vi "Keithley_Standalone_RS-232.vi"() -> ()   [LabVIEW 2013]
uses:
  subVIs/Current_Range_Control.ctl
  <vilib>/Utility/file.llb/Write To Spreadsheet File (DBL).vi
panel:
  out "Scan Number":i32
  in  "Current Range Ch 2":T1 items=["Autorange", "+/- 20 mikroA", "+/- 2 mikroA", "+/- 200 nA", "+/- 20 nA", "+/- 2 nA"]
  in  "Current Range Ch 1":T1 items=["Autorange", "+/- 20 mikroA", "+/- 2 mikroA", "+/- 200 nA", "+/- 20 nA", "+/- 2 nA"]
  out "Standard Error":dbl[](array[numeric])
  in  "1D Array Order":i32[](array[numeric])
  out "Chart 2":cluster{"Time Array OUT":dbl[], dbl[]}(graph)
  out "Chart 1":cluster{"Time Array OUT":dbl[], dbl[]}(graph)
  in  "Invert Ch 2":bool
  in  "Invert Ch 1":bool
  out "t_loop":u32
  out "dumped data (%)":dbl
  out "dumped data":i32
  in  "Cluster":T2={"Baudrate (9600)"=57600, "Data Bits (8)"=8, "Parity (None)"=0, "Stop Bits (1)"=10, "Flow Control (None)"=0, "End Mode for Reads (TermChar)"=2} {"End Mode for Reads (TermChar)" items=["None", "Last Bit", "TermChar"]; "Flow Control (None)" items=["None", "XON/XOFF", "RTS/CTS", "XON/XOFF & RTS/CTS", "DTR/DSR", "XON/XOFF & DTR/DSR"]; "Stop Bits (1)" items=["1.0"=10, "1.5"=15, "2.0"=20]; "Parity (None)" items=["None", "Odd", "Even", "Mark", "Space"]; "Baudrate (9600)" items=["300"=300, "600"=600, "1200"=1200, "2400"=2400, "4800"=4800, "9600"=9600, "19200"=19200, "38400"=38400, "57600"=57600, "115200"=115200]}
  in  "VISA resource name":refnum<visa-resource-name>="COM1"
  out "SD Keithley":dbl[](array[numeric])
  out "Mean Keithley":dbl[](array[numeric])
  out "buffer":string
  out "use data":bool
  out "Status":i32 format="%.0b"
  in  "Stop Keithley":bool
  in  "error in (no error)":errorcluster
  out "error out":errorcluster
  # "file structure:     column 1      column 2       column 3\n                              time (s)         Ch 1 (amp)     Ch 2 (amp)"
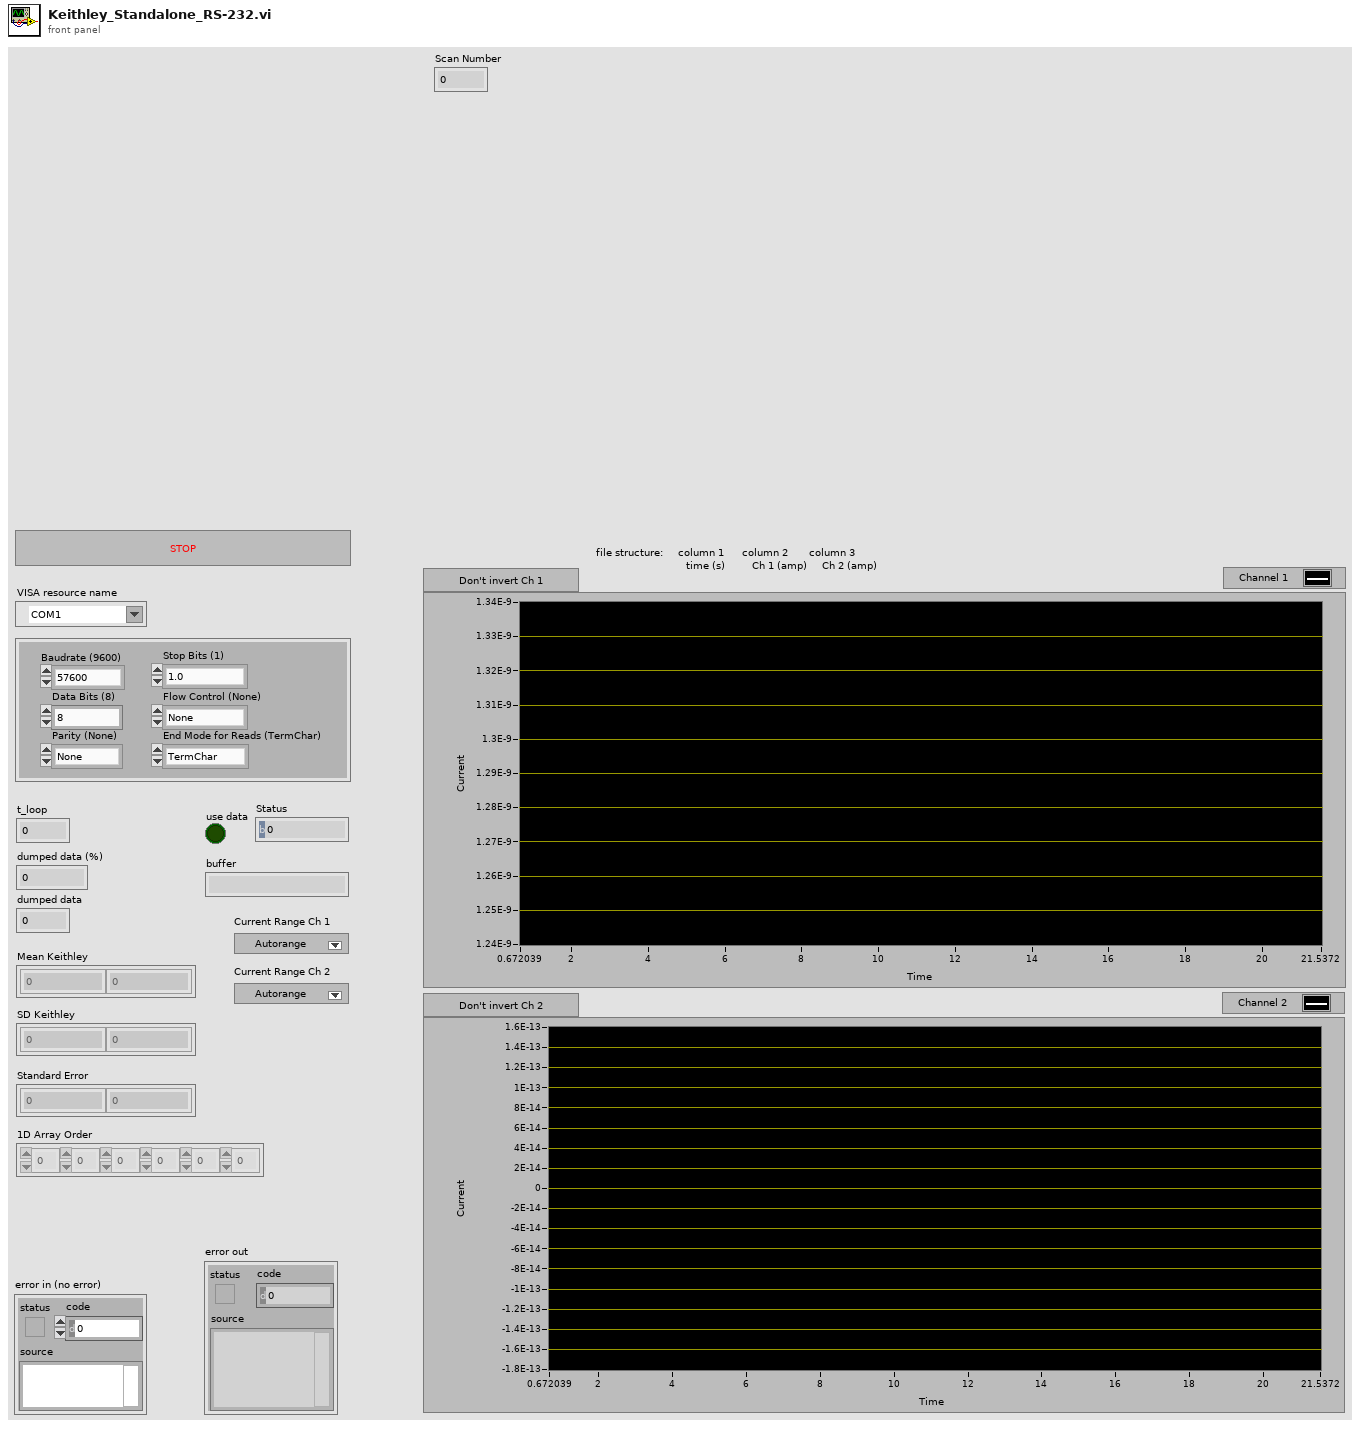
[diagram p1: front panel]
types:
  T1 = typedef "Current_Range_Control.ctl" = u16
  T2 = cluster{"Baudrate (9600)":u32, "Data Bits (8)":u16, "Parity (None)":u16, "Stop Bits (1)":u16, "Flow Control (None)":u16, "End Mode for Reads (TermChar)":u16}
  T3 = cluster{"Time Array OUT":dbl[], "Array OUT":dbl[]}
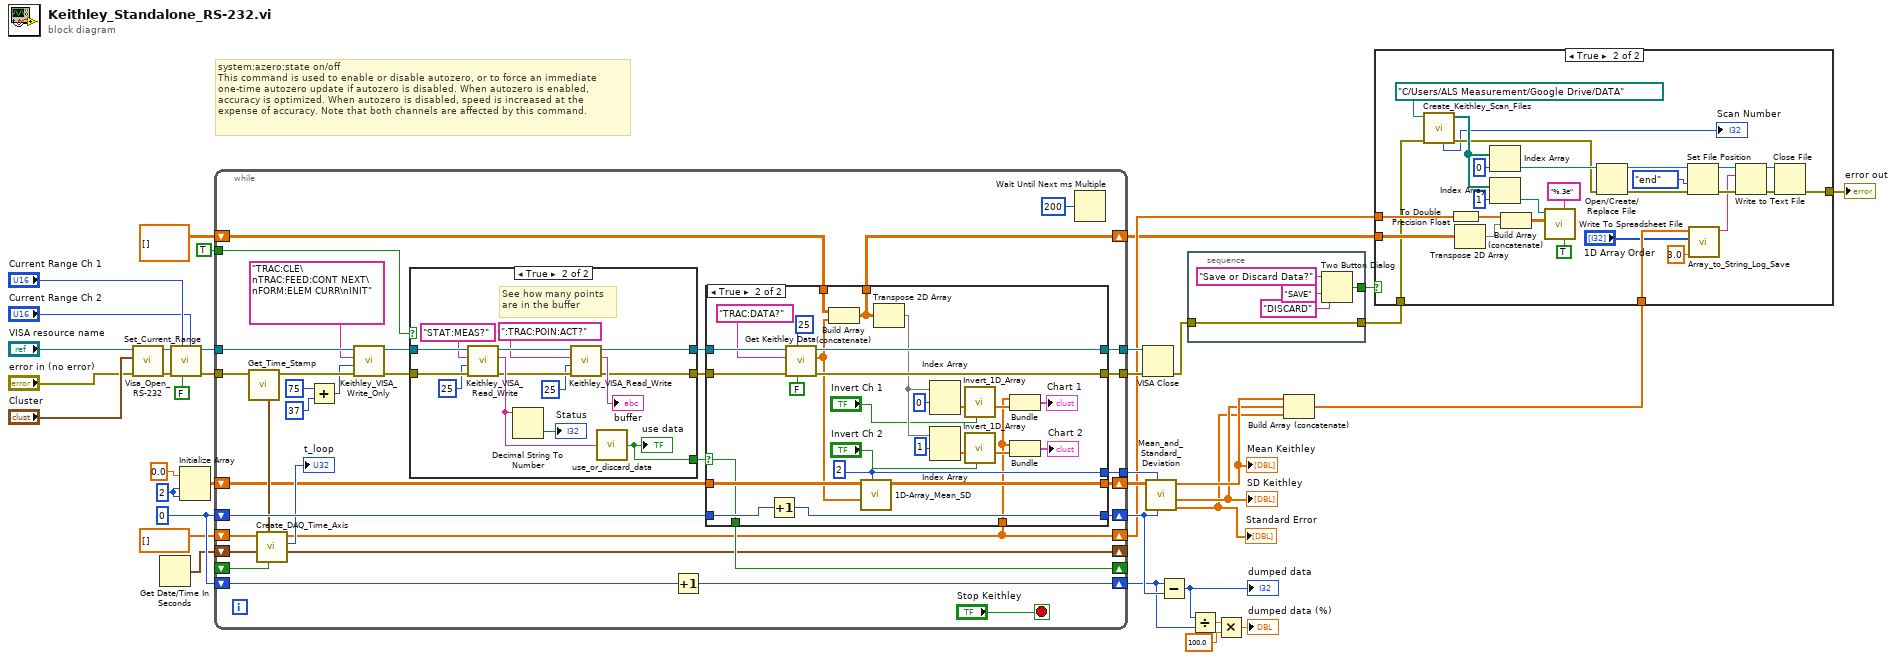
[diagram p0: block diagram]
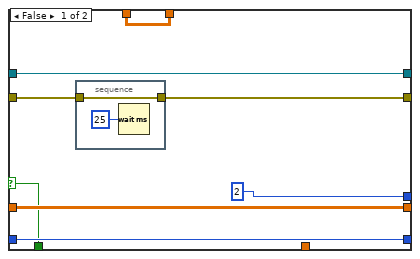
[diagram p3: hidden frame]
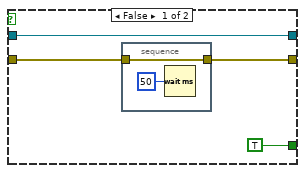
[diagram p4: hidden frame]
diagram:
  w24 = 0
  w37 = 2 ("dimension size")
  # "system:azero:state on/off\nThis command is used to enable or disable autozero, or to force an immediate\none-time autozero update if autozero is disabled. When autozero is enabled,\naccuracy is optimized. When autozero is disabled, speed is increased at the\nexpense of accuracy. Note that both channels are affected by this command."
  n1 = call "Visa_Open_RS-232.vi"("error in (no error)"="error in (no error)", "Cluster"="Cluster", "ComPort"="VISA resource name") -> ("error out"=w17:errorcluster, "VISA resource name out"=w15:refnum<visa-resource-name>)  [unwired: 7 in]
  n2 = Get Date/Time In Seconds() -> (seconds since 1Jan1904=w23:timestamp)
  n3 = call "Set_Current_Range.vi"("Current Range Ch 2"="Current Range Ch 2", "GPIB (t) / RS-232 (f)"=FALSE, "Current Range Ch 1"="Current Range Ch 1", "error in (no error)"=w17, "VISA resource name"=w15) -> ("error out"=w16:errorcluster, "VISA resource name out"=w18:refnum<visa-resource-name>)  [unwired: 5 in]
  n4 = Initialize Array(0.0 ("element"), w37, w37) -> (w36:dbl[][])
  n5 = while {
    tunnel: w18 -> [w61]
    tunnel: w16 -> [w55]
    tunnel: [w72] -> w20
    tunnel: [w56] -> w21
    tunnel: TRUE ("Check Completeness of Data (true)") -> [w71]
    shift-right: [w69] -> w34
    shift-left: w36 -> [w43]
    tunnel: [w68] -> w35
    shift-right: [w66] -> w30
    shift-left: w24 -> [w67]
    shift-right: [w63] -> w28
    shift-left: w24 -> [w64]
    shift-right: [w40] -> w9
    shift-left: dbl[] [] ("Time Array OUT") -> [w52]
    shift-right: [w41] -> w8
    shift-left: dbl[][] [] -> [w42]
    shift-right: [w50] -> _
    shift-left: w23 -> [w51]
    shift-right: [w53] -> _
    shift-left: _ -> [w49]
    stop <- "Stop Keithley" stop-if-true
    n6 = call "Get_Time_Stamp.vi"("error in"=w55) -> ("error out"=w54:errorcluster, "current time"=w47:timestamp)  [unwired: 9 in]
    n7 = call "Create_DAQ_Time_Axis.vi"("NOT [Last Data Point Dumped?]"=w49, "Time Stamp Current Iteration"=w47, "Time Stamp Last Iteration"=w51, "Time Array IN"=w52) -> ("Time Stamp Current Iteration"=w50:timestamp, "Loop Time (ms)"=→"t_loop":u32, "Time Array OUT"=w40:dbl[])  [unwired: 5 in]
    n8 = Add(x=u32 75 ("milliseconds to wait"), y=u32 37) -> (x+y=w45:u32)
    n9 = call "Keithley_VISA_Write_Only.vi"("error in (no error)"=w54, "milliseconds to wait"=w45, "command"="TRAC:CLE\nTRAC:FEED:CONT NEXT\nFORM:ELEM CURR\nINIT", "VISA resource name"=w61) -> ("error out"=w59:errorcluster, "VISA resource name out"=w60:refnum<visa-resource-name>)  [unwired: 6 in]
    n10 = case shown="True" w71 {
      tunnel: w60 -> [w114 w128]
      tunnel: w59 -> [w112 w129]
      tunnel: [w114 w119] -> w70
      tunnel: [TRUE w117] -> w62
      tunnel: [w111 w118] -> w65
      frame False {
        n11 = stacked-sequence {
          tunnel: w112 -> [w116]
          tunnel: [w116] -> w111
          frame #0 {
            n12 = Wait (ms)(milliseconds to wait=u32 50) -> ()  [unwired: 1 out]
          }
        }
      }
      frame True {
        # "See how many points\nare in the buffer"
        n13 = call "Keithley_VISA_Read_Write.vi"("error in (no error)"=w129, "milliseconds to wait"=u32 25, "command"="STAT:MEAS?" ("write buffer"), "VISA resource name"=w128) -> ("error out"=w124:errorcluster, "read buffer"=w125:string, "VISA resource name out"=w123:refnum<visa-resource-name>)  [unwired: 5 in]
        n14 = Decimal String To Number(string=w125) -> (number=→"Status":i32)  [unwired: 2 in, 1 out]
        n15 = call "Keithley_VISA_Read_Write.vi"("error in (no error)"=w124, "milliseconds to wait"=u32 25, "command"=":TRAC:POIN:ACT?" ("write buffer"), "VISA resource name"=w123) -> ("error out"=w118:errorcluster, "read buffer"=→"buffer":string, "VISA resource name out"=w119:refnum<visa-resource-name>)  [unwired: 5 in]
        n16 = call "use_or_discard_data.vi"("Status"=w125) -> ("use data"=w117:bool)
        "use data" <- w117
      }
    }
    n17 = Increment(x=w64) -> (x+1=w63:i32)
    n18 = case shown="True" w62 {
      selector: w62 -> [w73 w98]
      tunnel: [w77 w108] -> w72
      tunnel: [w75 w107] -> w56
      tunnel: w70 -> [w77 w110]
      tunnel: w65 -> [w76 w109]
      tunnel: w43 -> [w80 w106]
      tunnel: [w80 w105] -> w69
      tunnel: [2 ("N") w104] -> w68
      tunnel: w67 -> [w78 w103]
      tunnel: [w78 w102] -> w66
      tunnel: [w74 w95] -> w41
      tunnel: w42 -> [w74 w99]
      tunnel: [w73 w98] -> w53
      tunnel: w40 -> [_ w84]
      frame False {
        n19 = stacked-sequence {
          tunnel: w76 -> [w82]
          tunnel: [w82] -> w75
          frame #0 {
            n20 = Wait (ms)(milliseconds to wait=u32 25) -> ()  [unwired: 1 out]
          }
        }
      }
      frame True {
        w104 = 2 ("N")
        n21 = Increment(x=w103) -> (x+1=w102:i32)
        n22 = call "Get Keithley Data.vi"("GPIB = true, RS-232 = false"=FALSE, "wait after write (ms)"=u32 25 ("milliseconds to wait"), "error in (no error)"=w109, "Command"="TRAC:DATA?", "VISA resource name"=w110) -> ("error out"=w107:errorcluster, "Data"=w97:dbl[], "VISA resource name out"=w108:refnum<visa-resource-name>)  [unwired: 3 in, 1 out]
        n23 = Build Array (concatenate)(w99, w97) -> (w95:dbl[][])
        n24 = call "1D-Array_Mean_SD.vi"("N"=w104, "Data Array"=w97, "IN"=w106) -> ("OUT"=w105:dbl[][])  [unwired: 8 in]
        n25 = Transpose 2D Array(2D array=w95) -> (transposed array=w96:dbl[][])
        n26 = Index Array(array=w96, index (row)=0 ("index")) -> (element=w91:dbl[])  [unwired: 1 in]
        n27 = Index Array(array=w96, index (row)=1 ("index")) -> (element=w92:dbl[])  [unwired: 1 in]
        n28 = call "Invert_1D_Array.vi"("Invert?"="Invert Ch 1", "Array IN"=w91) -> ("Array OUT"=w86:dbl[])  [unwired: 9 in]
        n29 = call "Invert_1D_Array.vi"("Invert?"="Invert Ch 2", "Array IN"=w92) -> ("Array OUT"=w85:dbl[])  [unwired: 9 in]
        n30 = Bundle("Time Array OUT"=w84, "Array OUT"=w86) -> (→"Chart 1":T3)  [unwired: 1 in]
        n31 = Bundle("Time Array OUT"=w84, "Array OUT"=w85) -> (→"Chart 2":T3)  [unwired: 1 in]
      }
    }
    n32 = Wait Until Next ms Multiple(millisecond multiple=u32 200) -> ()  [unwired: 1 out]
  }
  n33 = VISA Close(VISA resource name=w20, error in (no error)=w21) -> (error out=w3:errorcluster)
  n34 = call "Mean_and_Standard_Deviation.vi"("Iterations"=w30, "Data Points"=w35, "2D array"=w34) -> ("Standard Error"=w11:dbl[], "Standard Deviation"=w12:dbl[], "Mean"=w13:dbl[])  [unwired: 6 in]
  "Mean Keithley" <- w13
  "SD Keithley" <- w12
  "Standard Error" <- w11
  n35 = Subtract(x=w28, y=w30) -> (x-y=w29:i32)
  "dumped data" <- w29
  n36 = stacked-sequence {
    tunnel: [w135] -> w1
    tunnel: w3 -> [w131]
    tunnel: [w131] -> w2
    frame #0 {
      n37 = Two Button Dialog(message="Save or Discard Data?", 1:"DISCARD" ("F button name (\"Cancel\")"), 2:"SAVE" ("T button name (\"OK\")")) -> (T button?=w135:bool)
    }
  }
  n38 = Divide(x=w29, y=w28) -> (x/y=w27:dbl)
  n39 = Multiply(x=w27, y=100.0) -> (x*y=→"dumped data (%)":dbl)
  n40 = Build Array (concatenate)(w13, w12, w11) -> (w10:dbl[])
  n41 = case shown="True" w1 {
    tunnel: w10 -> [_ w164]
    tunnel: w9 -> [_ w156]
    tunnel: w8 -> [_ w155]
    tunnel: [w136 w138] -> w4
    tunnel: w2 -> [w136 w137]
    frame False {
    }
    frame True {
      n42 = call "Create_Keithley_Scan_Files.vi"("error in (no error)"=w137, "base path"=path "C:/Users/ALS Measurement/Google Drive/DATA" ("file path (use dialog)")) -> ("error out"=w149:errorcluster, "Save Files Array"=w161:path[], "Scan Number"=→"Scan Number":i32)  [unwired: 5 in, 2 out]
      n43 = To Double Precision Float(number=w156) -> (double precision float=w158:dbl[])
      n44 = Transpose 2D Array(2D array=w155) -> (transposed array=w157:dbl[][])
      n45 = Index Array(array=w161, index=0) -> (element=w152:path)
      n46 = Index Array(array=w161, index=1) -> (element=w160:path)
      n47 = Build Array (concatenate)(w158, w157) -> (w159:dbl[][])
      n48 = call-poly <vilib>:"Write To Spreadsheet File.vi"("transpose? (no:F)"=TRUE, "format (%.3f)"="%.3e", "2D data"=w159, "file path (dialog if empty)"=w160) -> ()  [unwired: 4 in, 1 out]
      n49 = Open/Create/Replace File(file path (use dialog)=w152, error in=w149) -> (refnum out=w146:refnum<file>, error out=w148:errorcluster)  [unwired: 4 in, 1 out]
      n50 = Set File Position(refnum=w146, from (0:start)=enum16{"start", "end", "current"}."end", error in=w148) -> (refnum out=w145:refnum<file>, error out=w144:errorcluster)  [unwired: 1 in]
      n51 = call "Array_to_String_Log_Save.vi"("Precision (6)"=3.0, "1D Array Order"="1D Array Order", "1D Array"=w164) -> ("Save String"=w141:string)  [unwired: 7 in, 1 out]
      n52 = Write to Text File(file (use dialog)=w145, text=w141, error in=w144) -> (refnum out=w143:refnum<file>, error out=w142:errorcluster)  [unwired: 1 in, 1 out]
      n53 = Close File(refnum=w143, error in=w142) -> (error out=w138:errorcluster)  [unwired: 1 out]
    }
  }
  "error out" <- w4
